vi "test_RPLiDAR_Main6 grid-map.vi"() -> ()   [LabVIEW 2019]
uses:
  Ctrl/system_hw.ctl
  Ctrl/cmd_common.ctl
  Ctrl/rplidar_cmd.ctl
  <vilib>/Analysis/Matrix/Numeric/Conversions/Array To Matrix - RA2.vi
  <vilib>/Analysis/Matrix/NI_Matrix.lvlib
panel:
  in  "tab":enum32{"메인", "설정"}(tab)
  out "dt":u32=4
  out "n queue":i32
  in  "limit_ptn":u8=5
  in  "limit_len":dbl=0.2
  out "buff chart":u32(graph)=65886
  out "xy graph":T1(graph)
  in  "xy_resolution":dbl=0.02
  in  "EXTEND_AREA":dbl=1.0
  out "Occupacy Grid Map":dbl[][](graph)
  in  "map y size":u32
  in  "map x size":u32
  in  "map y center":u32
  in  "map x center":u32
  in  "HW info":T2={"AGV"=enum."none", "Lidar 1"=enum."RPLidar A3", "Lidar 2"=enum."none", "GPS"=enum."none", "Camera"=enum."none", "Joystick"=enum."none", "sound"=enum."none", "IMU"=enum."none", "Led"=enum."none"}
  in  "RPLidar cfg":T3={"port"="COM8", "dt"=4, "update n"=50, "speed"=444, "rate "=256000} {"speed" scale=100.0..1000.0}
  out "r-theta":cluster{"angle":dbl, "distance":dbl}[](array[cluster])=[{"angle"=59.46875, "distance"=339.5}, {"angle"=60.28125, "distance"=339.5}, {"angle"=60.953125, "distance"=339.5}, {"angle"=61.765625, "distance"=339.5}, {"angle"=62.859375, "distance"=339.0}, {"angle"=63.671875, "distance"=336.5}, {"angle"=67.921875, "distance"=326.5}, {"angle"=68.609375, "distance"=327.5}, {"angle"=92.96875, "distance"=320.0}, {"angle"=94.078125, "distance"=325.0}, {"angle"=94.890625, "distance"=323.5}, {"angle"=95.578125, "distance"=325.0}, {"angle"=96.390625, "distance"=330.0}, {"angle"=97.5, "distance"=340.0}, {"angle"=98.3125, "distance"=346.0}, {"angle"=98.765625, "distance"=346.0}, {"angle"=99.828125, "distance"=351.5}, {"angle"=100.6875, "distance"=348.5}, {"angle"=0.0, "distance"=0.0}, {"angle"=28.484375, "distance"=350.0}, {"angle"=29.546875, "distance"=344.0}, {"angle"=31.453125, "distance"=340.5}, {"angle"=32.265625, "distance"=334.5}, {"angle"=34.875, "distance"=326.5}, {"angle"=48.484375, "distance"=328.5}, {"angle"=55.03125, "distance"=347.0}]
  out "clustering":cluster{"X":dbl, "Y":dbl}[](graph)
  in  "stop":bool=TRUE
  # "RPLidar Occupancy Grid Map Tester"
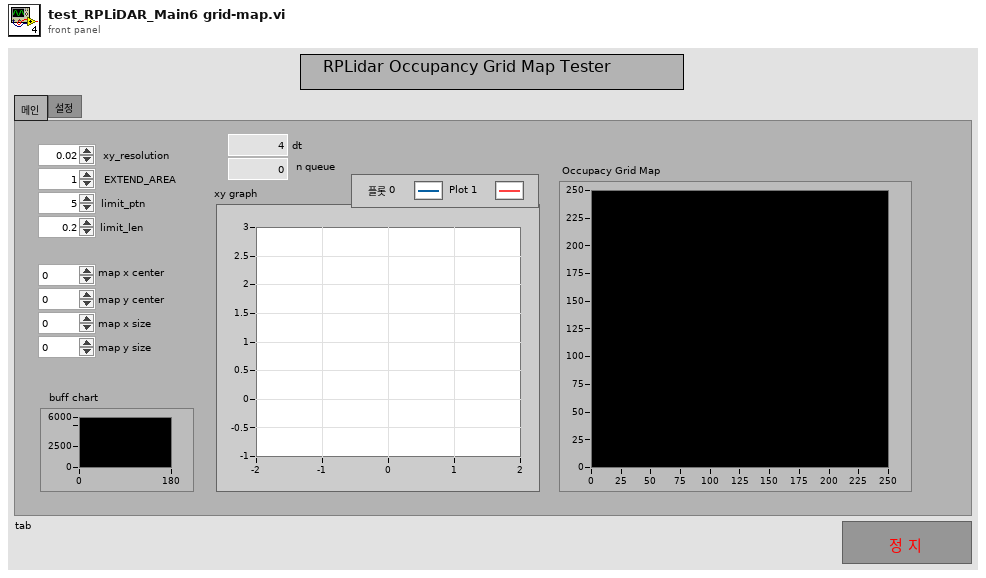
[diagram p1: front panel]
types:
  T1 = cluster{"clustering":cluster{"X":dbl, "Y":dbl}[]}[]
  T2 = typedef "system_hw.ctl" = cluster{"AGV":enum16{"none", "ERP42", "Scout", "Ycar"}, "Lidar 1":enum16{"none", "VLP16", "TIM571", "RPLidar A2", "RPLidar A3"}, "Lidar 2":enum16{"none", "VLP16", "TIM571", "RPLidar A2", "RPLidar A3"}, "GPS":enum16{"none", "F9P", "M8P", "PwrPak7", "19X HVS"}, "Camera":enum16{"none", "C920", "C922", "GT1290C", "MS LifeCam"}, "Joystick":enum16{"none", "joystick"}, "sound":enum16{"none", "speaker"}, "IMU":enum16{"none", "MW-AHRSv1"}, "Led":enum16{"none", "LedMatrix 8x32"}}
  T3 = cluster{"port":refnum<visa-resource-name>, "dt":u32, "update n":u8, "speed":u16, "rate ":u32}
  T4 = typedef "cmd_common.ctl" = enum16{"read", "write"}
  T5 = typedef "NI_Matrix.lvlib/RealMatrix.ctl" = dbl[][]
  T6 = cluster{"xy_resolution":dbl, "EXTEND_AREA":dbl, "MAX_RANGE":dbl, "NP":u32, "NTh":u32, "Q":T5, "R":T5, "Q_sim":T5, "R_sim":T5, "rf_id":cluster{"x":dbl, "y":dbl}[], "map x size":u32, "map y size":u32, "map x center":u32, "map y center":u32}
  T7 = cluster{"xy array out":cluster{"x":dbl, "y":dbl}[]}
  T8 = cluster{"clustering":cluster{"X":dbl, "Y":dbl}[]}
  T9 = cluster{"ox":dbl[], "oy":dbl[], "occupancy map":T5, "x_true":T5, "u":T5, "z":T5, "PEst":T5, "min x":dbl, "min y":dbl, "max x":dbl, "max y":dbl, "yw":i32, "xw":i32, "center x":i32, "center y":i32}
  T10 = typedef "rplidar_cmd.ctl" = enum16{"init", "health", "spin", "scan", "read", "stop", "close"}
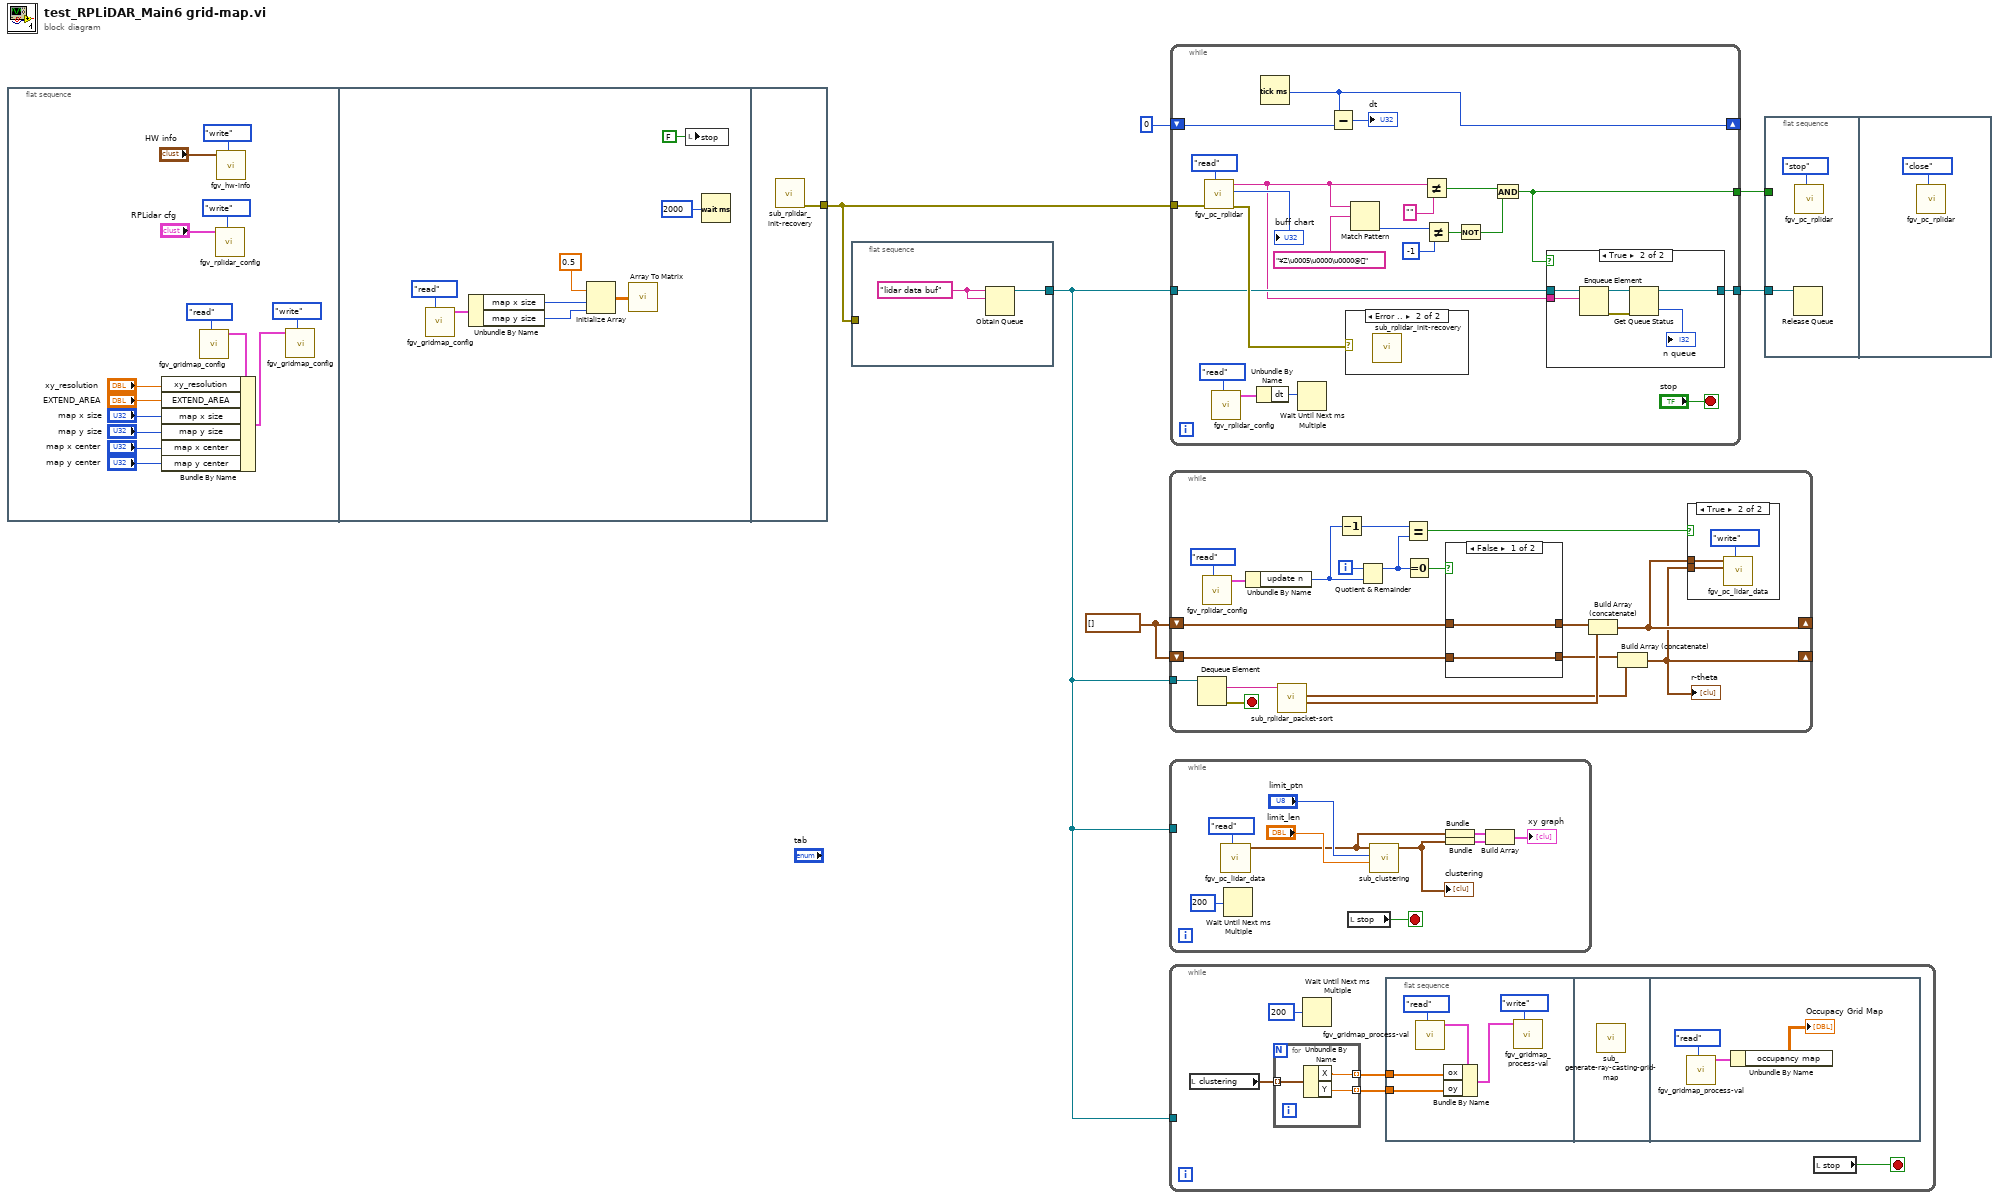
[diagram p0: block diagram]
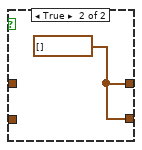
[diagram p3: hidden frame]
diagram:
  w3 = cluster{dbl, dbl}[] []
  n1 = flat-sequence {
    tunnel: [w29] -> w2
    frame #0 {
      n2 = call "fgv_gridmap_config.vi"("cmd"=cmd_common."read") -> ("pf-val out"=w14:T6)  [unwired: 10 in]
      n3 = Bundle By Name(cluster=w14, "xy_resolution"="xy_resolution", "EXTEND_AREA"="EXTEND_AREA", "map x size"="map x size", "map y size"="map y size", "map x center"="map x center", "map y center"="map y center") -> (w12:T6)
      n4 = call "fgv_rplidar_config.vi"("cmd"=enum16{"read", "write"}."write", "RPLidar cfg"="RPLidar cfg") -> ()  [unwired: 8 in, 2 out]
      n5 = call "fgv_hw-info.vi"("cmd"=enum16{"write", "read"}."write", "HW info"="HW info") -> ()  [unwired: 9 in, 1 out]
      n6 = call "fgv_gridmap_config.vi"("cmd"=cmd_common."write", "pf-val"=w12) -> ()  [unwired: 9 in, 1 out]
    }
    frame #1 {
      n7 = call "fgv_gridmap_config.vi"("cmd"=cmd_common."read") -> ("pf-val out"=w23:T6)  [unwired: 10 in]
      n8 = Unbundle By Name(w23) -> ("map x size"=w22:u32, "map y size"=w21:u32)
      n9 = Initialize Array(0.5 ("원소"), w22, w21) -> (w25:dbl[][])
      n10 = call-poly <vilib>:"Array To Matrix.vi"("Real 2D Array"=w25) -> ()  [unwired: 1 out]
      n11 = local write "stop"(FALSE ("stop")) -> ()
      n12 = Wait (ms)(milliseconds to wait=u32 2000) -> ()  [unwired: 1 out]
    }
    frame #2 {
      n13 = call "sub_rplidar_init-recovery.vi"() -> ("error out"=w29:errorcluster)  [unwired: 11 in]
    }
  }
  n14 = flat-sequence {
    tunnel: [w30] -> w1
    tunnel: w2 -> [_]
    frame #0 {
      w31 = "lidar data buf" ("name (unnamed)")
      n15 = Obtain Queue(name (unnamed)=w31, element data type=w31) -> (queue out=w30:refnum<queue>)  [unwired: 3 in, 2 out]
    }
  }
  n16 = while {
    shift-right: [w33] -> _
    shift-left: w3 -> [w47]
    tunnel: w1 -> [w50]
    shift-right: [w32] -> _
    shift-left: w3 -> [w35]
    i -> [w46]
    stop <- w39 stop-if-true
    n17 = Dequeue Element(queue=w50) -> (element=w49:string, error out=w39:errorcluster)  [unwired: 2 in, 2 out]
    n18 = call "fgv_rplidar_config.vi"("cmd"=enum16{"read", "write"}."read") -> ("RPLidar cfg out"=w42:T3)  [unwired: 9 in, 1 out]
    n19 = Unbundle By Name(w42) -> ("update n"=w41:u8)
    n20 = call "sub_rplidar_packet-sort.vi"("rplidar data str"=w49) -> ("xydata"=w44:cluster{"x":dbl, "y":dbl}[], "angle-distance"=w34:cluster{"angle":dbl, "distance":dbl}[])  [unwired: 8 in, 1 out]
    n21 = Decrement(x=w41) -> (x-1=w37:u8)
    n22 = Quotient & Remainder(x=w46, y=w41) -> (x-y*floor(x/y)=w38:i32)  [unwired: 1 out]
    n23 = Equal?(x=w37, y=w38) -> (x = y?=w40:bool)
    n24 = Equal To 0?(x=w38) -> (x = 0?=w45:bool)
    n25 = case shown="False" w45 {
      tunnel: [w55 w56] -> w48
      tunnel: w47 -> [w55 _]
      tunnel: [w54 w56] -> w36
      tunnel: w35 -> [w54 _]
      frame False {
      }
      frame True {
        w56 = cluster{dbl, dbl}[] []
      }
    }
    n26 = Build Array (concatenate)(w48, w44) -> (w33:cluster{"x":dbl, "y":dbl}[])
    n27 = Build Array (concatenate)(w36, w34) -> (w32:cluster{"angle":dbl, "distance":dbl}[])
    "r-theta" <- w32
    n28 = case shown="True" w40 {
      tunnel: w33 -> [_ w52]
      tunnel: w32 -> [_ w51]
      frame False {
      }
      frame True {
        n29 = call "fgv_pc_lidar_data.vi"("cmd"=enum16{"init", "read", "write"}."write", "rtheta array"=w51, "xy array"=w52) -> ()  [unwired: 7 in, 2 out]
      }
    }
  }
  n30 = while {
    tunnel: w1 -> [_]
    stop <- w66 stop-if-true
    n31 = call "fgv_pc_lidar_data.vi"("cmd"=enum16{"init", "read", "write"}."read") -> ("xy array out"=w61:cluster{"x":dbl, "y":dbl}[])  [unwired: 9 in, 1 out]
    n32 = Wait Until Next ms Multiple(millisecond multiple=u32 200) -> ()  [unwired: 1 out]
    n33 = local read "stop"() -> (w66:bool)
    n34 = call "sub_clustering.vi"("limit_len"="limit_len", "limit_ptn"="limit_ptn", "2d data"=w61) -> ("clustering"=w60:cluster{"X":dbl, "Y":dbl}[])  [unwired: 8 in]
    "clustering" <- w60
    n35 = Bundle("xy array out"=w61) -> (w58:T7)  [unwired: 1 in]
    n36 = Bundle("clustering"=w60) -> (w59:T8)  [unwired: 1 in]
    n37 = Build Array(w58, w59) -> (→"xy graph":T1)
  }
  n38 = while {
    tunnel: w1 -> [_]
    stop <- w71 stop-if-true
    n39 = local read "clustering"() -> (w69:cluster{"X":dbl, "Y":dbl}[])
    n40 = for {
      tunnel: w69 -> [w83] mode=indexing
      tunnel: [w82] -> w68 mode=indexing
      tunnel: [w81] -> w67 mode=indexing
      n41 = Unbundle By Name(w83) -> ("X"=w82:dbl, "Y"=w81:dbl)
    }
    n42 = Wait Until Next ms Multiple(millisecond multiple=u32 200) -> ()  [unwired: 1 out]
    n43 = flat-sequence {
      tunnel: w68 -> [w73]
      tunnel: w67 -> [w72]
      frame #0 {
        n44 = call "fgv_gridmap_process-val.vi"("cmd"=cmd_common."read") -> ("p-val  2"=w76:T9)  [unwired: 10 in]
        n45 = Bundle By Name(cluster=w76, "ox"=w73, "oy"=w72) -> (w77:T9)
        n46 = call "fgv_gridmap_process-val.vi"("cmd"=cmd_common."write", "p-val"=w77) -> ()  [unwired: 9 in, 1 out]
      }
      frame #1 {
        n47 = call "sub_generate-ray-casting-grid-map.vi"() -> ()  [unwired: 12 in]
      }
      frame #2 {
        n48 = call "fgv_gridmap_process-val.vi"("cmd"=cmd_common."read") -> ("p-val  2"=w80:T9)  [unwired: 10 in]
        n49 = Unbundle By Name(w80) -> ("occupancy map"=→"Occupacy Grid Map":T5)
      }
    }
    n50 = local read "stop"() -> (w71:bool)
  }
  n51 = while {
    tunnel: w2 -> [w104]
    shift-right: [w91] -> _
    shift-left: u32 0 ("millisecond timer value") -> [w92]
    tunnel: [w86] -> w5
    tunnel: w1 -> [w87]
    tunnel: [w84] -> w4
    stop <- "stop" stop-if-true
    n52 = call "fgv_pc_rplidar.vi"("cmd"=rplidar_cmd."read", "error in"=w104) -> ("error out"=w93:errorcluster, "serial buf"=→"buff chart":u32, "read buffer"=w85:string)  [unwired: 7 in]
    n53 = call "fgv_rplidar_config.vi"("cmd"=enum16{"read", "write"}."read") -> ("RPLidar cfg out"=w95:T3)  [unwired: 9 in, 1 out]
    n54 = Unbundle By Name(w95) -> ("dt"=w94:u32)
    n55 = Tick Count (ms)() -> (millisecond timer value=w91:u32)
    n56 = Wait Until Next ms Multiple(millisecond multiple=w94) -> ()  [unwired: 1 out]
    n57 = Subtract(x=w91, y=w92) -> (x-y=→"dt":u32)
    n58 = case shown="Error .." w93 {
      frame No Error {
      }
      frame Error {
        n59 = call "sub_rplidar_init-recovery.vi"() -> ()  [unwired: 11 in, 1 out]
      }
    }
    n60 = Match Pattern(string=w85, regular expression="¥Z\u0005\u0000\u0000@") -> (offset past match=w103:i32)  [unwired: 1 in, 3 out]
    n61 = Not Equal?(x=w85, y="") -> (x != y?=w97:bool)
    n62 = Not Equal?(x=w103, y=-1) -> (x != y?=w100:bool)
    n63 = Not(x=w100) -> (.not. x?=w98:bool)
    n64 = And(x=w97, y=w98) -> (x .and. y?=w86:bool)
    n65 = case shown="True" w86 {
      tunnel: w87 -> [w106 w112]
      tunnel: [w106 w109] -> w84
      tunnel: w85 -> [_ w110]
      frame False {
      }
      frame True {
        n66 = Enqueue Element(queue=w112, element=w110) -> (queue out=w111:refnum<queue>, error out=w108:errorcluster)  [unwired: 2 in, 1 out]
        n67 = Get Queue Status(queue=w111, error in (no error)=w108) -> (queue out=w109:refnum<queue>, # elements in queue=→"n queue":i32)  [unwired: 1 in, 6 out]
      }
    }
  }
  n68 = flat-sequence {
    tunnel: w5 -> [_]
    tunnel: w4 -> [w113]
    frame #0 {
      n69 = Release Queue(queue=w113) -> ()  [unwired: 2 in, 3 out]
      n70 = call "fgv_pc_rplidar.vi"("cmd"=rplidar_cmd."stop") -> ()  [unwired: 8 in, 3 out]
    }
    frame #1 {
      n71 = call "fgv_pc_rplidar.vi"("cmd"=rplidar_cmd."close") -> ()  [unwired: 8 in, 3 out]
    }
  }
